vi "Get Process Class Actions.vi"(8 "error in (no error)":errorcluster {"code" format="Error %.0f"}, 11 "VIDoc Printer In":refnum<class "VIDoc Printer.lvclass">) -> (0 "error out":errorcluster {"code" format="Error %.0f"}, 2 "Process Class Actions":T1[](array[typedef]), 3 "VIDoc Printer Out":refnum<class "VIDoc Printer.lvclass">)   [LabVIEW 2023, in "VIDoc Printer.lvlib" / "VIDoc Printer.lvclass"]
uses:
  VIDoc Printer.lvclass
  Controls/Process Class Enum.ctl
  VIDoc Printer.lvclass/VIDoc Printer.ctl
  Get Class Settings - Memory.vi
  Get Class Settings - By Folder.vi
  Get Class Settings - By Tree.vi
  Get Class Settings - By List.vi
  Get Class Settings - List Detail Level.vi
  Get Class Settings - Details.vi
  Get Class Settings - Detail Options - Description.vi
  Get Class Settings - Detail Options - Properties.vi
  Get Class Settings - Detail Options - Inheritance.vi
  Get Class Settings - Inheritance Options - Parent Classes.vi
  Get Class Settings - Inheritance Options - Parent Interfaces.vi
  Get Class Settings - Inheritance Options - Parent Libraries.vi
  Get Class Settings - Inheritance Options - Friends.vi
  Get Class Settings - CPD Detail Level.vi
  Get Class Settings - Methods Detail Level.vi
  Get Class Settings - Get Accessor Detail Level.vi
  Get Class Settings - Set Accessor Detail Level.vi
  Get Class Settings - Controls Detail Level.vi
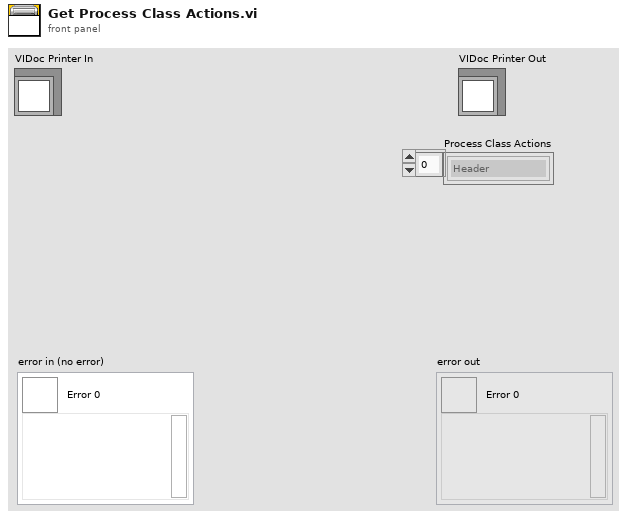
[diagram p1: front panel]
types:
  T1 = typedef "VIDoc Printer.lvlib/VIDoc Printer.lvclass/Process Class Enum.ctl" = enum16{"Header", "Memory", "By Folder", "By Tree", "By List", "Description", "Properties", "Inheritance", "Inheritance Classes", "Inheritance Interfaces", "Inheritance Libraries", "Friends", "Class Private Data", "Methods", "Get Accessors", "Set Accessors", "Controls"}
  T2 = typedef "VIDoc Printer.lvlib/Printer Settings.lvclass/Detail Level Enum.ctl" = enum16{"None", "Minimal", "Standard", "Full"}
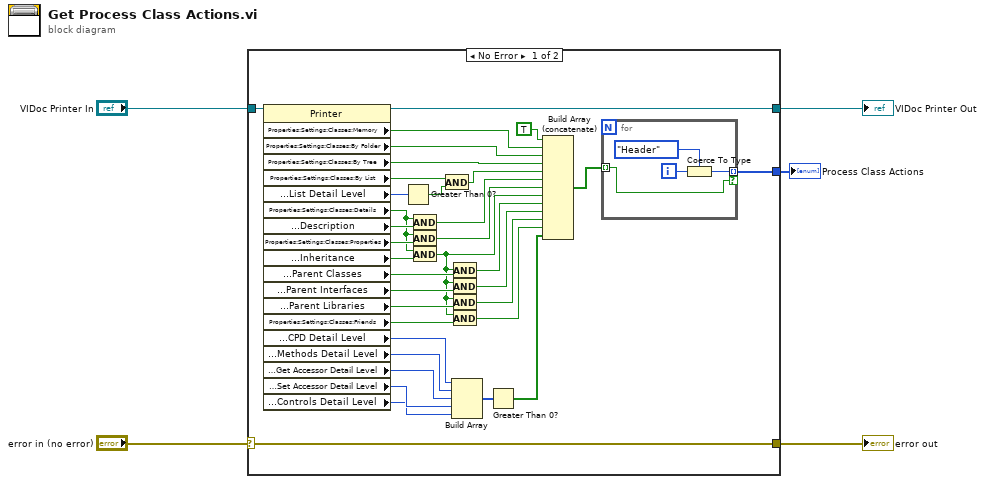
[diagram p0: block diagram]
diagram:
  n1 = case shown="No Error" "error in (no error)" {
    selector: "error in (no error)" -> [w40 w46]
    tunnel: [w40 w46] -> w4
    tunnel: [w26 w45] -> w2
    tunnel: "VIDoc Printer In" -> [w27 w45]
    tunnel: [w24 _] -> w1
    frame No Error {
      n2 = property class="Printer"(reference=w27) -> (reference out=w26:refnum<class "VIDoc Printer.lvclass">, "Properties:Settings:Classes:Memory"=w31:bool, "Properties:Settings:Classes:By Folder"=w30:bool, "Properties:Settings:Classes:By Tree"=w29:bool, "Properties:Settings:Classes:By List"=w28:bool, "Properties:Settings:Classes:List Detail Level"=w23:T2, "Properties:Settings:Classes:Details"=w16:bool, "Properties:Settings:Classes:Description"=w20:bool, "Properties:Settings:Classes:Properties"=w18:bool, "Properties:Settings:Classes:Inheritance"=w15:bool, "Properties:Settings:Classes:Parent Classes"=w14:bool, "Properties:Settings:Classes:Parent Interfaces"=w13:bool, "Properties:Settings:Classes:Parent Libraries"=w12:bool, "Properties:Settings:Classes:Friends"=w11:bool, "Properties:Settings:Classes:CPD Detail Level"=w37:T2, "Properties:Settings:Classes:Methods Detail Level"=w36:T2, "Properties:Settings:Classes:Get Accessor Detail Level"=w38:T2, "Properties:Settings:Classes:Set Accessor Detail Level"=w35:T2, "Properties:Settings:Classes:Controls Detail Level"=w34:T2)  [unwired: 1 in, 1 out]
      n3 = Greater Than 0?(x=w23) -> (x > 0?=w21:bool)
      n4 = And(x=w16, y=w20) -> (x .and. y?=w19:bool)
      n5 = And(x=w16, y=w18) -> (x .and. y?=w17:bool)
      n6 = And(x=w16, y=w15) -> (x .and. y?=w10:bool)
      n7 = And(x=w28, y=w21) -> (x .and. y?=w22:bool)
      n8 = And(x=w10, y=w14) -> (x .and. y?=w9:bool)
      n9 = And(x=w10, y=w13) -> (x .and. y?=w8:bool)
      n10 = And(x=w10, y=w12) -> (x .and. y?=w7:bool)
      n11 = And(x=w10, y=w11) -> (x .and. y?=w6:bool)
      n12 = Build Array(w37, w36, w38, w35, w34) -> (w33:T2[])
      n13 = Greater Than 0?(x=w33) -> (x > 0?=w39:bool[])
      n14 = Build Array (concatenate)(TRUE ("element"), w31, w30, w29, w22, w19, w17, w10, w9, w8, w7, w6, w39) -> (w25:bool[])
      n15 = for {
        tunnel: w25 -> [w44] mode=indexing
        tunnel: [w41] -> w24 mode=indexing if=w44
        i -> [w43]
        n16 = Coerce To Type(0:w43, 1:Process_Class_Enum."Header") -> (2:w41:T1)
      }
    }
    frame Error {
    }
  }
  "error out" <- w4
  "VIDoc Printer Out" <- w2
  "Process Class Actions" <- w1
